vi "Initialize.vi"(8 "error in (no error)":errorcluster, 11 "NI-XNET CAN Writer Execution Unit in":refnum<class "NI-XNET CAN Writer Execution Unit.lvclass">) -> (0 "error out":errorcluster, 3 "NI-XNET CAN Writer Execution Unit out":refnum<class "NI-XNET CAN Writer Execution Unit.lvclass">)   [LabVIEW 2020, in "Communication Bus Template Engine.lvlib" / "Implementation.lvlib" / "NI-XNET CAN Writer Execution Unit.lvclass"]
uses:
  NI-XNET CAN Writer Execution Unit.lvclass
  NI-XNET CAN Writer Execution Unit.lvclass/NI-XNET CAN Writer Execution Unit.ctl
  <vilib>/xnet/xnet.llb/XNET Create Session (Signal Output Single-point).vi
  <resource>/objmgr/xnet.rc
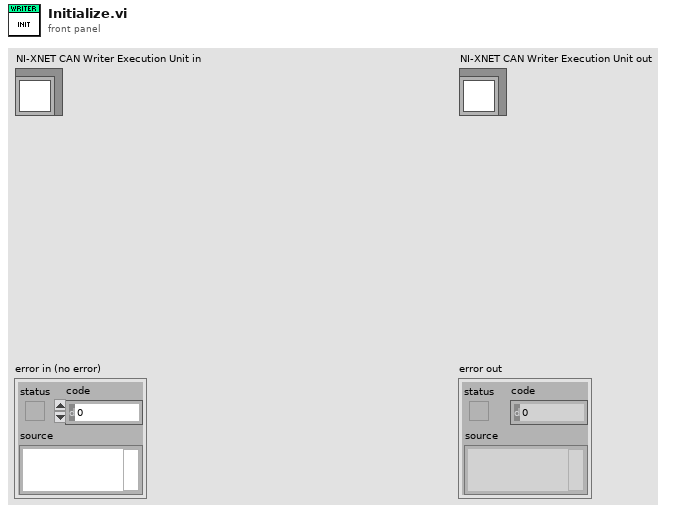
[diagram p1: front panel]
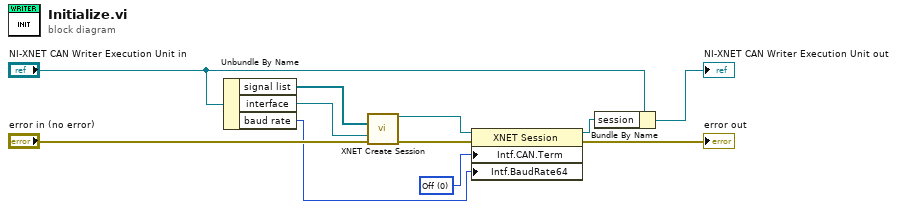
[diagram p0: block diagram]
diagram:
  w10 = u32 0 items=["Off", "On"] ("Interface:CAN:Termination")
  n1 = Unbundle By Name("NI-XNET CAN Writer Execution Unit in") -> ("signal list"=w6:refnum<k21>[], "interface"=w5:refnum<k21>, "baud rate"=w1:u64)
  n2 = call-poly <vilib>:"XNET Create Session.vi"("signal list"=w6, "interface"=w5, "error in (no error)"="error in (no error)") -> ("session out"=w11:refnum<k21>, "error out"=w9:errorcluster)  [unwired: 11 in]
  n3 = property class="XNET Session"(reference=w11, error in=w9, "Intf.CAN.Term"=w10, "Intf.BaudRate64"=w1) -> (reference out=w2:refnum<k21>, error out=→"error out":errorcluster)
  n4 = Bundle By Name(cluster="NI-XNET CAN Writer Execution Unit in", "session"=w2) -> (→"NI-XNET CAN Writer Execution Unit out":refnum<class "NI-XNET CAN Writer Execution Unit.lvclass">)
